vi "trigger.vi"(8 "error in (no error)":errorcluster, 11 "Modbus in":refnum<class "Modbus.lvclass">) -> (0 "error out":errorcluster, 3 "Modbus out":refnum<class "Modbus.lvclass">)   [LabVIEW 2016, in "RTModbusFPGA.lvlib" / "Modbus.lvclass"]
uses:
  Modbus.lvclass
  Modbus.lvclass/Modbus.ctl
  Common_RT_FPGA/IBooleanControl/IBooleanControl.lvclass
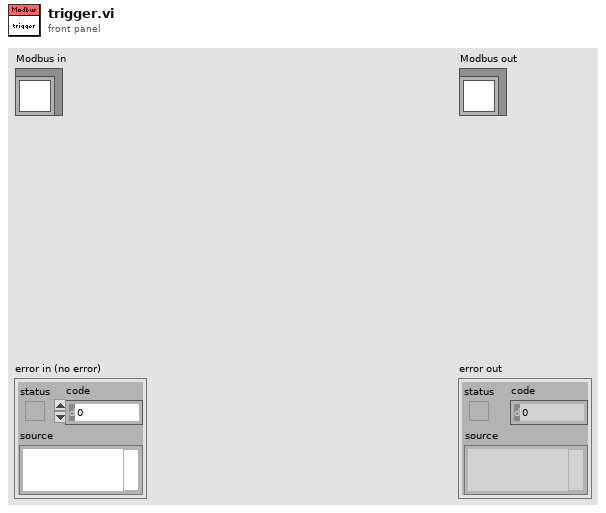
[diagram p1: front panel]
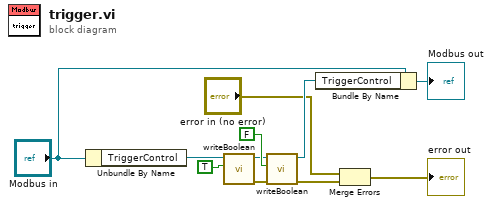
[diagram p0: block diagram]
diagram:
  n1 = Unbundle By Name("Modbus in") -> ("TriggerControl"=w7:refnum<class "IBooleanControl.lvclass">)
  n2 = call-dynamic "writeBoolean.vi"("Data"=TRUE, "IBooleanControl in"=w7) -> ("error out"=w4:errorcluster, "IBooleanControl out"=w6:refnum<class "IBooleanControl.lvclass">)  [unwired: 8 in]
  n3 = call-dynamic "writeBoolean.vi"("error in (no error)"=w4, "Data"=FALSE, "IBooleanControl in"=w6) -> ("error out"=w3:errorcluster, "IBooleanControl out"=w5:refnum<class "IBooleanControl.lvclass">)  [unwired: 7 in]
  n4 = Bundle By Name(cluster="Modbus in", "TriggerControl"=w5) -> (→"Modbus out":refnum<class "Modbus.lvclass">)
  n5 = Merge Errors("error in (no error)", w3) -> (→"error out":errorcluster)
